vi "VII Slave Read Bytes.vi"(7 "pLen":u16, 8 "error in (no error)":errorcluster, 9 "I2CIndex":i32, 10 "DevIndex":i32, 11 "DevType":i32) -> (0 "error out":errorcluster, 2 "function return":i32, 3 "pReadData":string, 5 "pLen out":u16)   [LabVIEW 2012, in "ControlI2C.lvlib"]
doc: "int __stdcall VII_SlaveReadBytes(int DevType,int DevIndex,int I2CIndex,unsigned char* pReadData,unsigned short *pLen);"
uses:
  ControlI2C.lvlib
  Ginkgo_Driver.dll
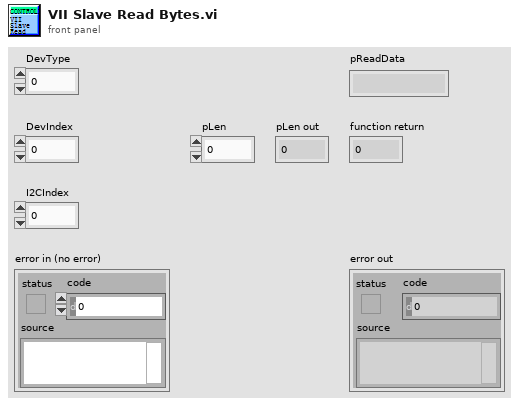
[diagram p1: front panel]
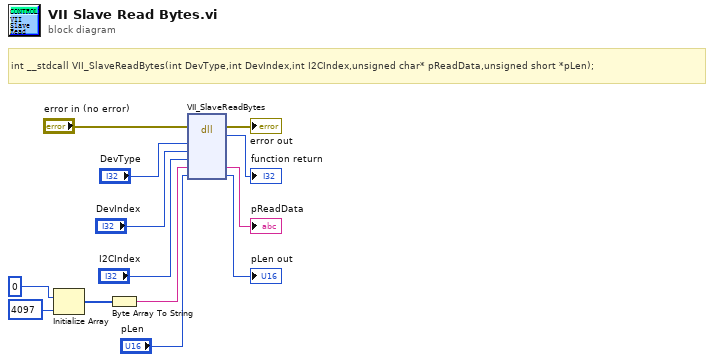
[diagram p0: block diagram]
diagram:
  # "int __stdcall VII_SlaveReadBytes(int DevType,int DevIndex,int I2CIndex,unsigned char* pReadData,unsigned short *pLen);"
  n1 = Initialize Array(u8 0 ("element"), 4097 ("dimension size")) -> (w9:u8[])
  n2 = Byte Array To String(unsigned byte array=w9) -> (string=w8:string)
  n3 = dll-call lib="E:/Project/vt_ginkgo/truck/Ginkgo Driver/vs2010/Ginkgo_USB-I2C_API_v2.0.3.0/lib/labview_32bit/ControlI2C/Ginkgo_Driver.*" fn="VII_SlaveReadBytes"(error in="error in (no error)", "DevType"="DevType", "DevIndex"="DevIndex", "I2CIndex"="I2CIndex", "pReadData"=w8, "pLen"="pLen") -> (error out=→"error out":errorcluster, →"function return":i32, "pReadData"=→"pReadData":string, "pLen"=→"pLen out":u16)  [unwired: 5 in, 1 out]
